vi "seq analyse.vi"(0 "config":T1={"initialize"=enum."SR830", "6221"={"6221 Resource"="GPIB0::24::INSTR", "Delta status"=FALSE, "电流|RMS(A)"=0.0}, "SR830+6221"={"source"=0, "Current(A)"=0.0, "阻抗(Ohm)"=0.0, "SR830 1"=FALSE, "SR830 2"=FALSE, "SR830 3"=FALSE, "SR830 4"=FALSE, "VISA 1"="", "VISA 2"="", "VISA 3"="", "VISA 4"="", "Reserve 1"=-1, "Reserve 2"=-1, "Reserve 3"=-1, "Reserve 4"=-1, "Sensitivity 1"=-1, "Sensitivity 2"=-1, "Sensitivity 3"=-1, "Sensitivity 4"=-1, "量程入 1"=0, "量程入 2"=0, "量程入 3"=0, "量程入 4"=0}, "2400"={"2400"=FALSE, "VISA"="GPIB0::9::INSTR", "Output Level (0)"=1e-05, "Compliance  Level (0.1)"=10.0, "ch"=[]}, "ch"={"ch"=[], "current"=[], "change?"=[], "holding current\nwhen change ch?"=FALSE, "current offset"=[]}, "Instrument"={"limit"={"Field limit"=0.0, "Field rate limit"=0.0, "Temp limit"=0.0, "Temp low limit"=0.0, "Temp rate limit "=0.0}, "genarl"={"行数"=refnum, "编辑列表框？"=refnum, "列表框"=refnum, "camg 振荡状态"=refnum, "Aborting"=refnum, "数据文件"=refnum, "warning"=refnum, "vi路径"="", "Instrument Type"=enum."PPMS-Rotate"}, "cmag"={"TM620"="TCPIP0::192.168.1.5::4266::SOCKET", "M24C Resource"="GPIB0::24::INSTR", "4G supply"="", "Temp Status 24C"=refnum, "Temp"=refnum, "9T信号"=refnum, "4g supply status"=refnum, "in-plane"="", "out-plane"="", "in-plane signal"=FALSE, "out-plane signal"=FALSE, "in plane 信号"=refnum, "pzt volt"=refnum, "camg Rate"=refnum}, "lengtou2"={"750 visa"="", "750 rotate"="", "semaphore 340"=refnum, "semaphore 750"=refnum, "750 field status"=refnum, "Input (0:A) 340"=0, "340 Resource"="GPIB0::14::INSTR", "340 Status"=refnum, "Input (0:B) 340"=1, "Loop (0: 1)"=0, "Loop (1: 1)"=0, "TCP master instance"=refnum}, "lengtou"={"TCP master instance"=refnum, "335 Status"=refnum, "335 Resource "="GPIB0::24::INSTR", "Input (0:A) 335"=0, "Input (0:B) 335"=1, "Heater Output (1:1) 335"=1, "semaphore 335"=refnum}, "325 for test"={"quantum design"=refnum, "semaphore 325"=refnum, "325 Resource "="GPIB0::13::INSTR", "Input (0:A) 325"=0, "Heater Output (1:1) 325"=1, "325 Status"=refnum}}, "2614B"={"2614B chA"=FALSE, "2614B chB"=FALSE, "VISA"=""}, "33522b"={"33522b resource name"="GPIB0::16::INSTR", "零电压"=0.0, "最大电压"=148.0, "间隔"=4.0, "最小电压"=-48.0, "loop"=0.0, "压电陶瓷电压(Vpp)"=0.0}, "gating type"=enum."2614(daul)", "层数"=0, "行数"=0, "是否处理"=[], "current 2"=[], "StrainCell"={"RP100 resource name"="GPIB0::16::INSTR", "E4980 resource name"="GPIB0::16::INSTR", "RP100 Reset ?(True)"=TRUE, "Voltage1(V)"=0.0, "Voltage2(V)"=148.0, "interval"=4.0, "slew(V/s)"=-48.0}} {"Instrument"."325 for test"."Heater Output (1:1) 325" items=["1"=1, "2"=2]; "Instrument"."325 for test"."Input (0:A) 325" items=["A", "B"]; "Instrument"."lengtou"."Heater Output (1:1) 335" items=["1"=1, "2"=2]; "Instrument"."lengtou"."Input (0:B) 335" items=["A", "B"]; "Instrument"."lengtou"."Input (0:A) 335" items=["A", "B"]; "Instrument"."lengtou2"."Loop (1: 1)" items=["1", "2"]; "Instrument"."lengtou2"."Loop (0: 1)" items=["1", "2"]; "Instrument"."lengtou2"."Input (0:B) 340" items=["A", "B", "C", "D"]; "Instrument"."lengtou2"."Input (0:A) 340" items=["A", "B", "C", "D"]; "SR830+6221"."Sensitivity 4" items=["Auto Gain"=-1, "2 nV/fA"=0, "5 nV/fA"=1, "10 nV/fA"=2, "20 nV/fA"=3, "50 nV/fA"=4, "100 nV/fA"=5, "200 nV/fA"=6, "500 nV/fA"=7, "1 uV/pA"=8, "2 uV/pA"=9, "5 uV/pA"=10, "10 uV/pA"=11, "20 uV/pA"=12, "50 uV/pA"=13, "100 uV/pA"=14, "200 uV/pA"=15, "500 uV/pA"=16, "1 mV/nA"=17, "2 mV/nA"=18, "5 mV/nA"=19, "10 mV/nA"=20, "20 mV/nA"=21, "50 mV/nA"=22, "100 mV/nA"=23, "200 mV/nA"=24, "500 mV/mA"=25, "1 V/uA"=26]; "SR830+6221"."Sensitivity 3" items=["Auto Gain"=-1, "2 nV/fA"=0, "5 nV/fA"=1, "10 nV/fA"=2, "20 nV/fA"=3, "50 nV/fA"=4, "100 nV/fA"=5, "200 nV/fA"=6, "500 nV/fA"=7, "1 uV/pA"=8, "2 uV/pA"=9, "5 uV/pA"=10, "10 uV/pA"=11, "20 uV/pA"=12, "50 uV/pA"=13, "100 uV/pA"=14, "200 uV/pA"=15, "500 uV/pA"=16, "1 mV/nA"=17, "2 mV/nA"=18, "5 mV/nA"=19, "10 mV/nA"=20, "20 mV/nA"=21, "50 mV/nA"=22, "100 mV/nA"=23, "200 mV/nA"=24, "500 mV/mA"=25, "1 V/uA"=26]; "SR830+6221"."Sensitivity 1" items=["Auto Gain"=-1, "2 nV/fA"=0, "5 nV/fA"=1, "10 nV/fA"=2, "20 nV/fA"=3, "50 nV/fA"=4, "100 nV/fA"=5, "200 nV/fA"=6, "500 nV/fA"=7, "1 uV/pA"=8, "2 uV/pA"=9, "5 uV/pA"=10, "10 uV/pA"=11, "20 uV/pA"=12, "50 uV/pA"=13, "100 uV/pA"=14, "200 uV/pA"=15, "500 uV/pA"=16, "1 mV/nA"=17, "2 mV/nA"=18, "5 mV/nA"=19, "10 mV/nA"=20, "20 mV/nA"=21, "50 mV/nA"=22, "100 mV/nA"=23, "200 mV/nA"=24, "500 mV/mA"=25, "1 V/uA"=26]; "SR830+6221"."Sensitivity 2" items=["Auto Gain"=-1, "2 nV/fA"=0, "5 nV/fA"=1, "10 nV/fA"=2, "20 nV/fA"=3, "50 nV/fA"=4, "100 nV/fA"=5, "200 nV/fA"=6, "500 nV/fA"=7, "1 uV/pA"=8, "2 uV/pA"=9, "5 uV/pA"=10, "10 uV/pA"=11, "20 uV/pA"=12, "50 uV/pA"=13, "100 uV/pA"=14, "200 uV/pA"=15, "500 uV/pA"=16, "1 mV/nA"=17, "2 mV/nA"=18, "5 mV/nA"=19, "10 mV/nA"=20, "20 mV/nA"=21, "50 mV/nA"=22, "100 mV/nA"=23, "200 mV/nA"=24, "500 mV/mA"=25, "1 V/uA"=26]; "SR830+6221"."Reserve 4" items=["Auto Reserve"=-1, "High Reserve"=0, "Normal"=1, "Low Noise"=2]; "SR830+6221"."Reserve 3" items=["Auto Reserve"=-1, "High Reserve"=0, "Normal"=1, "Low Noise"=2]; "SR830+6221"."Reserve 2" items=["Auto Reserve"=-1, "High Reserve"=0, "Normal"=1, "Low Noise"=2]; "SR830+6221"."Reserve 1" items=["Auto Reserve"=-1, "High Reserve"=0, "Normal"=1, "Low Noise"=2]; "SR830+6221"."source" items=["SR830 1", "SR830 2", "SR830 3", "SR830 4"]}, 2 "数据队列":refnum<queue>, 3 "错误输入":errorcluster) -> (7 "config out":T1={"initialize"=enum."SR830", "6221"={"6221 Resource"="GPIB0::24::INSTR", "Delta status"=FALSE, "电流|RMS(A)"=0.0}, "SR830+6221"={"source"=0, "Current(A)"=0.0, "阻抗(Ohm)"=0.0, "SR830 1"=FALSE, "SR830 2"=FALSE, "SR830 3"=FALSE, "SR830 4"=FALSE, "VISA 1"="", "VISA 2"="", "VISA 3"="", "VISA 4"="", "Reserve 1"=-1, "Reserve 2"=-1, "Reserve 3"=-1, "Reserve 4"=-1, "Sensitivity 1"=-1, "Sensitivity 2"=-1, "Sensitivity 3"=-1, "Sensitivity 4"=-1, "量程入 1"=0, "量程入 2"=0, "量程入 3"=0, "量程入 4"=0}, "2400"={"2400"=FALSE, "VISA"="GPIB0::9::INSTR", "Output Level (0)"=1e-05, "Compliance  Level (0.1)"=10.0, "ch"=[]}, "ch"={"ch"=[], "current"=[], "change?"=[], "holding current\nwhen change ch?"=FALSE, "current offset"=[]}, "Instrument"={"limit"={"Field limit"=0.0, "Field rate limit"=0.0, "Temp limit"=0.0, "Temp low limit"=0.0, "Temp rate limit "=0.0}, "genarl"={"行数"=refnum, "编辑列表框？"=refnum, "列表框"=refnum, "camg 振荡状态"=refnum, "Aborting"=refnum, "数据文件"=refnum, "warning"=refnum, "vi路径"="", "Instrument Type"=enum."PPMS-Rotate"}, "cmag"={"TM620"="TCPIP0::192.168.1.5::4266::SOCKET", "M24C Resource"="GPIB0::24::INSTR", "4G supply"="", "Temp Status 24C"=refnum, "Temp"=refnum, "9T信号"=refnum, "4g supply status"=refnum, "in-plane"="", "out-plane"="", "in-plane signal"=FALSE, "out-plane signal"=FALSE, "in plane 信号"=refnum, "pzt volt"=refnum, "camg Rate"=refnum}, "lengtou2"={"750 visa"="", "750 rotate"="", "semaphore 340"=refnum, "semaphore 750"=refnum, "750 field status"=refnum, "Input (0:A) 340"=0, "340 Resource"="GPIB0::14::INSTR", "340 Status"=refnum, "Input (0:B) 340"=1, "Loop (0: 1)"=0, "Loop (1: 1)"=0, "TCP master instance"=refnum}, "lengtou"={"TCP master instance"=refnum, "335 Status"=refnum, "335 Resource "="GPIB0::24::INSTR", "Input (0:A) 335"=0, "Input (0:B) 335"=1, "Heater Output (1:1) 335"=1, "semaphore 335"=refnum}, "325 for test"={"quantum design"=refnum, "semaphore 325"=refnum, "325 Resource "="GPIB0::13::INSTR", "Input (0:A) 325"=0, "Heater Output (1:1) 325"=1, "325 Status"=refnum}}, "2614B"={"2614B chA"=FALSE, "2614B chB"=FALSE, "VISA"=""}, "33522b"={"33522b resource name"="GPIB0::16::INSTR", "零电压"=0.0, "最大电压"=148.0, "间隔"=4.0, "最小电压"=-48.0, "loop"=0.0, "压电陶瓷电压(Vpp)"=0.0}, "gating type"=enum."2614(daul)", "层数"=0, "行数"=0, "是否处理"=[], "current 2"=[], "StrainCell"={"RP100 resource name"="GPIB0::16::INSTR", "E4980 resource name"="GPIB0::16::INSTR", "RP100 Reset ?(True)"=TRUE, "Voltage1(V)"=0.0, "Voltage2(V)"=148.0, "interval"=4.0, "slew(V/s)"=-48.0}} {"Instrument"."325 for test"."Heater Output (1:1) 325" items=["1"=1, "2"=2]; "Instrument"."325 for test"."Input (0:A) 325" items=["A", "B"]; "Instrument"."lengtou"."Heater Output (1:1) 335" items=["1"=1, "2"=2]; "Instrument"."lengtou"."Input (0:B) 335" items=["A", "B"]; "Instrument"."lengtou"."Input (0:A) 335" items=["A", "B"]; "Instrument"."lengtou2"."Loop (1: 1)" items=["1", "2"]; "Instrument"."lengtou2"."Loop (0: 1)" items=["1", "2"]; "Instrument"."lengtou2"."Input (0:B) 340" items=["A", "B", "C", "D"]; "Instrument"."lengtou2"."Input (0:A) 340" items=["A", "B", "C", "D"]; "SR830+6221"."Sensitivity 4" items=["Auto Gain"=-1, "2 nV/fA"=0, "5 nV/fA"=1, "10 nV/fA"=2, "20 nV/fA"=3, "50 nV/fA"=4, "100 nV/fA"=5, "200 nV/fA"=6, "500 nV/fA"=7, "1 uV/pA"=8, "2 uV/pA"=9, "5 uV/pA"=10, "10 uV/pA"=11, "20 uV/pA"=12, "50 uV/pA"=13, "100 uV/pA"=14, "200 uV/pA"=15, "500 uV/pA"=16, "1 mV/nA"=17, "2 mV/nA"=18, "5 mV/nA"=19, "10 mV/nA"=20, "20 mV/nA"=21, "50 mV/nA"=22, "100 mV/nA"=23, "200 mV/nA"=24, "500 mV/mA"=25, "1 V/uA"=26]; "SR830+6221"."Sensitivity 3" items=["Auto Gain"=-1, "2 nV/fA"=0, "5 nV/fA"=1, "10 nV/fA"=2, "20 nV/fA"=3, "50 nV/fA"=4, "100 nV/fA"=5, "200 nV/fA"=6, "500 nV/fA"=7, "1 uV/pA"=8, "2 uV/pA"=9, "5 uV/pA"=10, "10 uV/pA"=11, "20 uV/pA"=12, "50 uV/pA"=13, "100 uV/pA"=14, "200 uV/pA"=15, "500 uV/pA"=16, "1 mV/nA"=17, "2 mV/nA"=18, "5 mV/nA"=19, "10 mV/nA"=20, "20 mV/nA"=21, "50 mV/nA"=22, "100 mV/nA"=23, "200 mV/nA"=24, "500 mV/mA"=25, "1 V/uA"=26]; "SR830+6221"."Sensitivity 1" items=["Auto Gain"=-1, "2 nV/fA"=0, "5 nV/fA"=1, "10 nV/fA"=2, "20 nV/fA"=3, "50 nV/fA"=4, "100 nV/fA"=5, "200 nV/fA"=6, "500 nV/fA"=7, "1 uV/pA"=8, "2 uV/pA"=9, "5 uV/pA"=10, "10 uV/pA"=11, "20 uV/pA"=12, "50 uV/pA"=13, "100 uV/pA"=14, "200 uV/pA"=15, "500 uV/pA"=16, "1 mV/nA"=17, "2 mV/nA"=18, "5 mV/nA"=19, "10 mV/nA"=20, "20 mV/nA"=21, "50 mV/nA"=22, "100 mV/nA"=23, "200 mV/nA"=24, "500 mV/mA"=25, "1 V/uA"=26]; "SR830+6221"."Sensitivity 2" items=["Auto Gain"=-1, "2 nV/fA"=0, "5 nV/fA"=1, "10 nV/fA"=2, "20 nV/fA"=3, "50 nV/fA"=4, "100 nV/fA"=5, "200 nV/fA"=6, "500 nV/fA"=7, "1 uV/pA"=8, "2 uV/pA"=9, "5 uV/pA"=10, "10 uV/pA"=11, "20 uV/pA"=12, "50 uV/pA"=13, "100 uV/pA"=14, "200 uV/pA"=15, "500 uV/pA"=16, "1 mV/nA"=17, "2 mV/nA"=18, "5 mV/nA"=19, "10 mV/nA"=20, "20 mV/nA"=21, "50 mV/nA"=22, "100 mV/nA"=23, "200 mV/nA"=24, "500 mV/mA"=25, "1 V/uA"=26]; "SR830+6221"."Reserve 4" items=["Auto Reserve"=-1, "High Reserve"=0, "Normal"=1, "Low Noise"=2]; "SR830+6221"."Reserve 3" items=["Auto Reserve"=-1, "High Reserve"=0, "Normal"=1, "Low Noise"=2]; "SR830+6221"."Reserve 2" items=["Auto Reserve"=-1, "High Reserve"=0, "Normal"=1, "Low Noise"=2]; "SR830+6221"."Reserve 1" items=["Auto Reserve"=-1, "High Reserve"=0, "Normal"=1, "Low Noise"=2]; "SR830+6221"."source" items=["SR830 1", "SR830 2", "SR830 3", "SR830 4"]}, 10 "错误输出":errorcluster)   [LabVIEW 2019, in "User lib.lvlib"]
uses:
  User lib.lvlib
  ctl/config.ctl
  <vilib>/NI/Modbus Library/API/Master/Modbus Master.lvclass
  ctl/initialize.ctl
  ctl/Instrument.ctl
  ctl/limit.ctl
  ctl/warning.ctl
  ctl/Instrument Type.ctl
  ctl/335 state.ctl
  ctl/9T mag field stauts.ctl
  C:/Users/fuyang/Desktop/postdoctor/labview/labview-measure/lib/QDInstrument.dll
  lib/QDInstrument.dll
  ctl/Gating type.ctl
  ctl/set type.ctl
  SubVI.lvlib
  Take Seq.lvlib
  9T cmag.lvlib
  Scan.lvlib
  nematic/Copy of StrainCell.lvlib
panel:
  out "step":string
  out "数值":i32
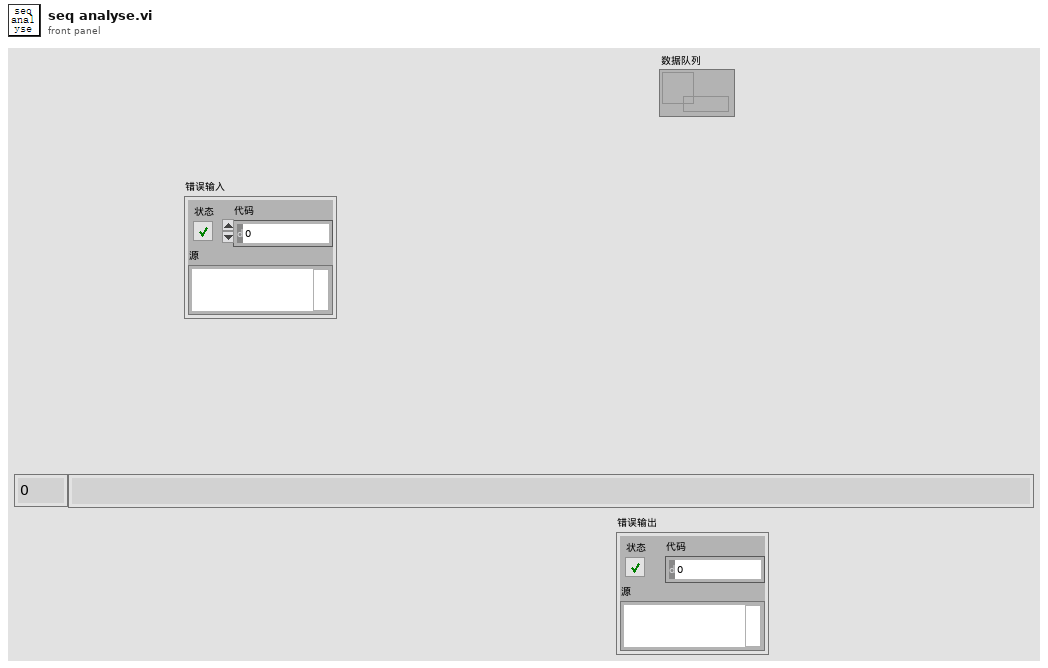
[diagram p1: front panel]
types:
  T1 = typedef "config.ctl" = cluster{"initialize":T2, "6221":cluster{"6221 Resource":refnum<visa-resource-name>, "Delta status":bool, "电流|RMS(A)":dbl}, "SR830+6221":cluster{"source":u16, "Current(A)":dbl, "阻抗(Ohm)":dbl, "SR830 1":bool, "SR830 2":bool, "SR830 3":bool, "SR830 4":bool, "VISA 1":refnum<visa-resource-name>, "VISA 2":refnum<visa-resource-name>, "VISA 3":refnum<visa-resource-name>, "VISA 4":refnum<visa-resource-name>, "Reserve 1":i16, "Reserve 2":i16, "Reserve 3":i16, "Reserve 4":i16, "Sensitivity 1":i16, "Sensitivity 2":i16, "Sensitivity 3":i16, "Sensitivity 4":i16, "量程入 1":i32, "量程入 2":i32, "量程入 3":i32, "量程入 4":i32}, "2400":cluster{"2400":bool, "VISA":refnum<visa-resource-name>, "Output Level (0)":dbl, "Compliance  Level (0.1)":dbl, "ch":i32[]}, "ch":cluster{"ch":i32[], "current":dbl[], "change?":bool[], "holding current\nwhen change ch?":bool, "current offset":dbl[]}, "Instrument":T3, "2614B":cluster{"2614B chA":bool, "2614B chB":bool, "VISA":refnum<visa-resource-name>}, "33522b":cluster{"33522b resource name":refnum<visa-resource-name>, "零电压":dbl, "最大电压":dbl, "间隔":dbl, "最小电压":dbl, "loop":dbl, "压电陶瓷电压(Vpp)":dbl}, "gating type":T7, "层数":i32, "行数":i32, "是否处理":bool[], "current 2":dbl[], "StrainCell":cluster{"RP100 resource name":refnum<visa-resource-name>, "E4980 resource name":refnum<visa-resource-name>, "RP100 Reset ?(True)":bool, "Voltage1(V)":dbl, "Voltage2(V)":dbl, "interval":dbl, "slew(V/s)":dbl}}
  T2 = typedef "initialize.ctl" = enum16{"SR830", "keithley6221-SR830", "Delta", "Delta-tunnelling", "keithley6221-2182-DC", "PZT", "StrainCell", "4200"}
  T3 = typedef "Instrument.ctl" = cluster{"limit":T4, "genarl":cluster{"行数":refnum<vi>, "编辑列表框？":refnum<vi>, "列表框":refnum<vi>, "camg 振荡状态":refnum<vi>, "Aborting":refnum<vi>, "数据文件":refnum<vi>, "warning":refnum<vi>, "vi路径":string, "Instrument Type":T5}, "cmag":cluster{"TM620":refnum<visa-resource-name>, "M24C Resource":refnum<visa-resource-name>, "4G supply":refnum<visa-resource-name>, "Temp Status 24C":refnum<vi>, "Temp":refnum<vi>, "9T信号":T6, "4g supply status":refnum<vi>, "in-plane":refnum<visa-resource-name>, "out-plane":refnum<visa-resource-name>, "in-plane signal":bool, "out-plane signal":bool, "in plane 信号":T6, "pzt volt":refnum<vi>, "camg Rate":refnum<vi>}, "lengtou2":cluster{"750 visa":refnum<visa-resource-name>, "750 rotate":refnum<visa-resource-name>, "semaphore 340":T6, "semaphore 750":T6, "750 field status":refnum<vi>, "Input (0:A) 340":u16, "340 Resource":refnum<visa-resource-name>, "340 Status":refnum<vi>, "Input (0:B) 340":u16, "Loop (0: 1)":u16, "Loop (1: 1)":u16, "TCP master instance":refnum<class "Modbus Master.lvclass">}, "lengtou":cluster{"TCP master instance":refnum<class "Modbus Master.lvclass">, "335 Status":refnum<vi>, "335 Resource ":refnum<visa-resource-name>, "Input (0:A) 335":u16, "Input (0:B) 335":u16, "Heater Output (1:1) 335":u16, "semaphore 335":T6}, "325 for test":cluster{"quantum design":refnum<k24>, "semaphore 325":T6, "325 Resource ":refnum<visa-resource-name>, "Input (0:A) 325":u16, "Heater Output (1:1) 325":u16, "325 Status":refnum<vi>}}
  T4 = typedef "limit.ctl" = cluster{"Field limit":dbl, "Field rate limit":dbl, "Temp limit":dbl, "Temp low limit":dbl, "Temp rate limit ":dbl}
  T5 = typedef "Instrument Type.ctl" = enum16{"PPMS", "VersaLab", "DynaCool", "SVSM", "PPMS-Rotate", "Lakeshore335", "lengtou2", "9T mag old", "9T cmag", "9T cmag DAC", "9T cmag rotate", "test"}
  T6 = typedef "Semaphore RefNum" = refnum<k1>
  T7 = typedef "Gating type.ctl" = enum32{"null", "2614(daul)", "2400", "6517B"}
  T8 = typedef "set type.ctl" = enum16{"temp", "field", "position", "gating", "current", "PZT", "StrainCell", "time"}
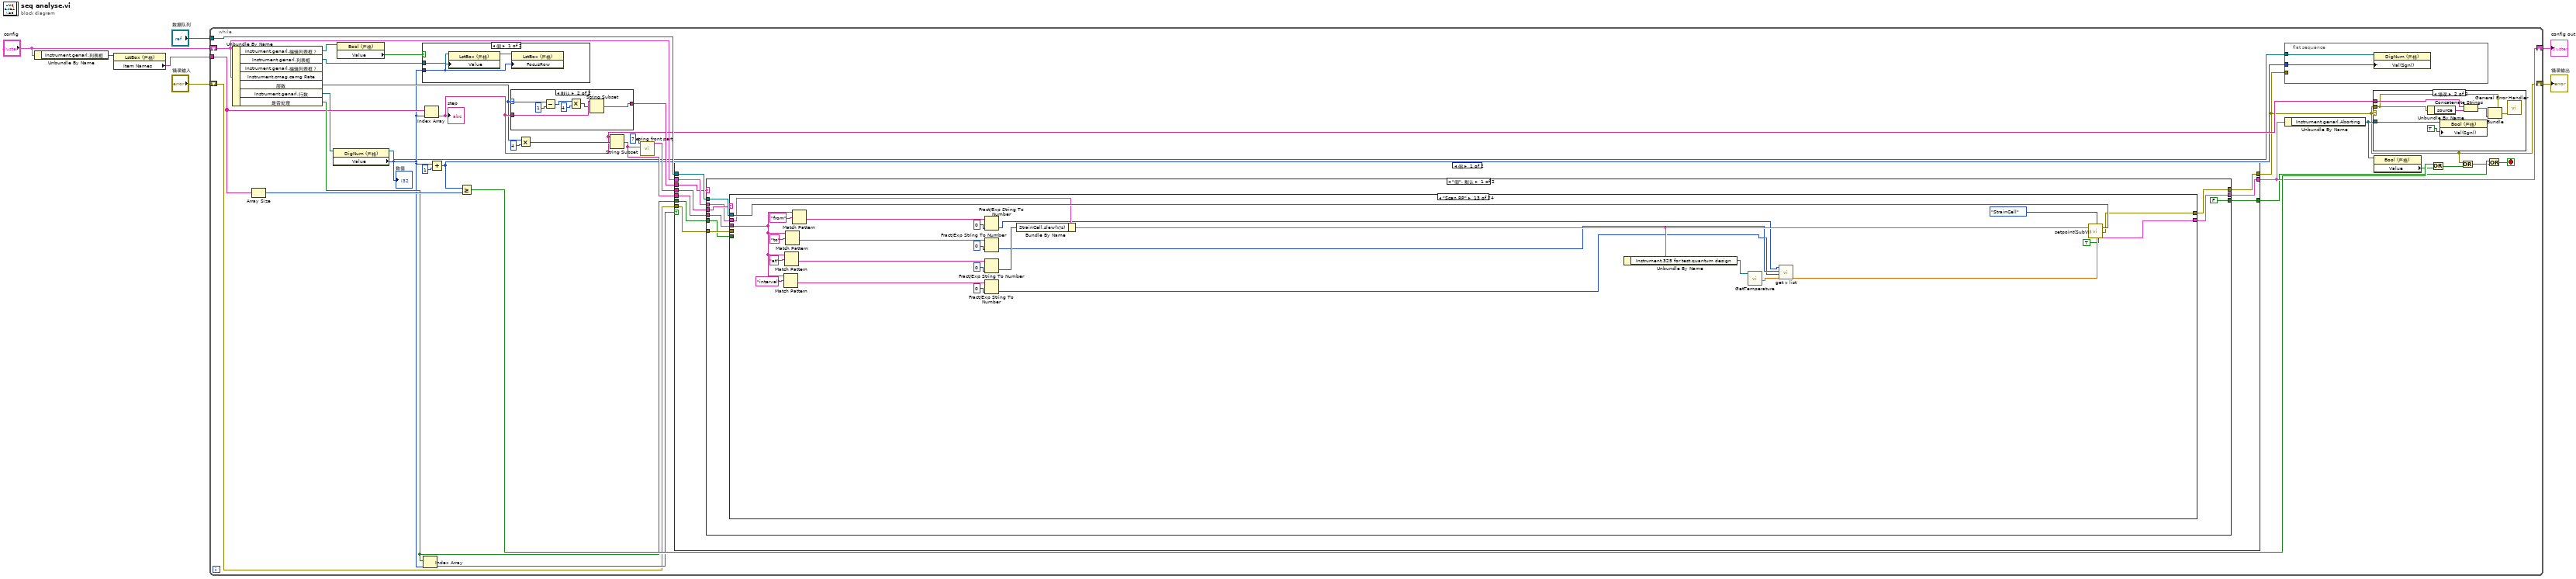
[diagram p0: block diagram]
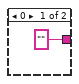
[diagram p2: hidden frame]
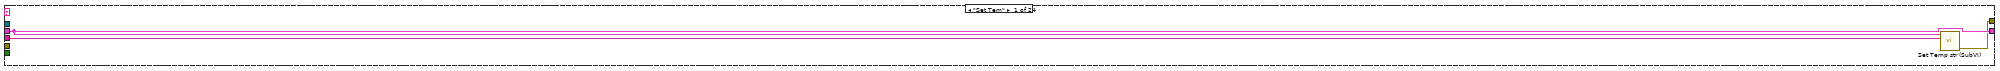
[diagram p5: hidden frame]
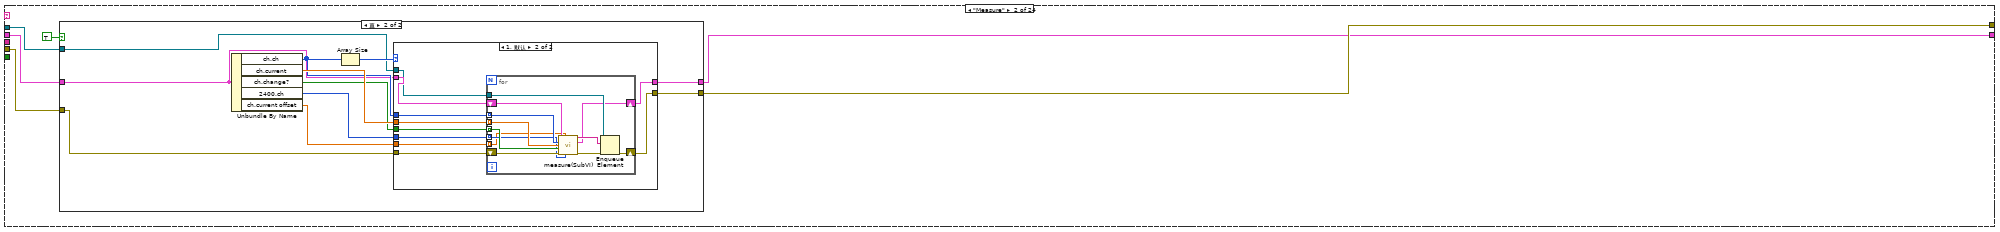
[diagram p6: hidden frame]
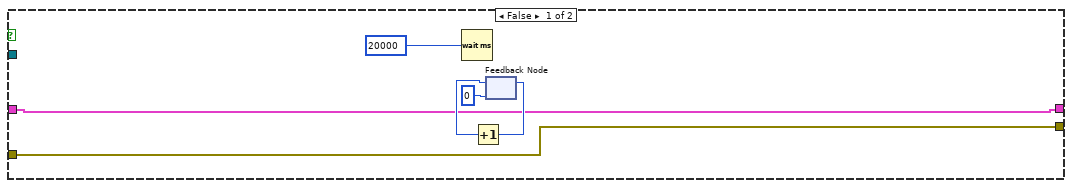
[diagram p7: hidden frame]
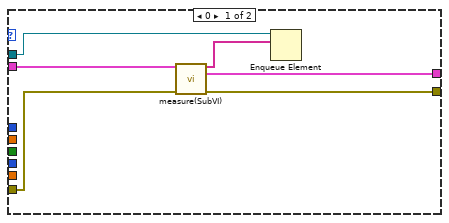
[diagram p8: hidden frame]
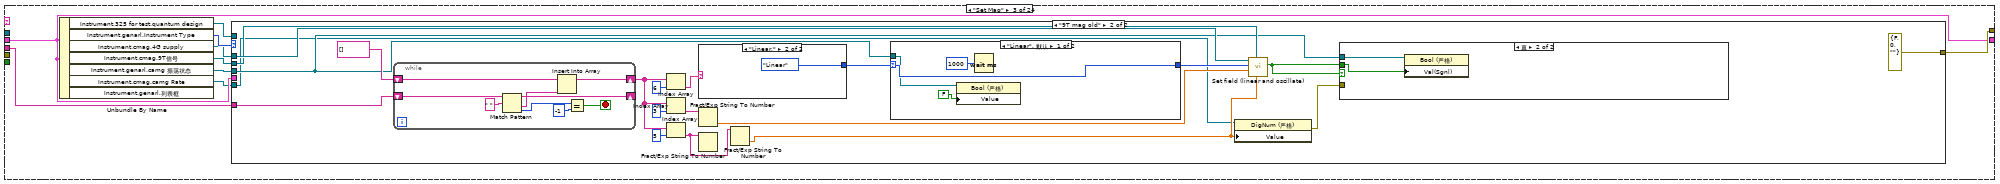
[diagram p9: hidden frame]
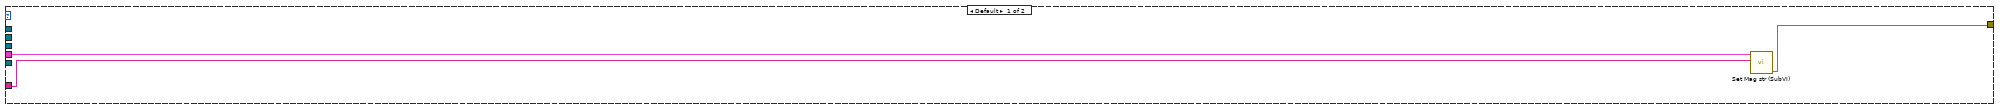
[diagram p10: hidden frame]
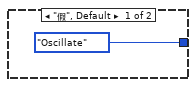
[diagram p13: hidden frame]
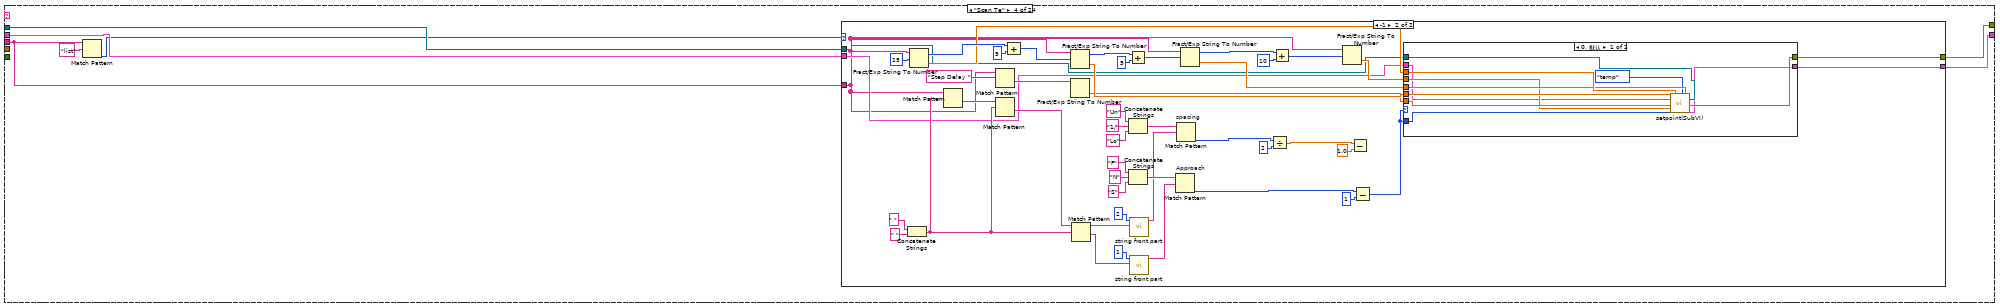
[diagram p14: hidden frame]
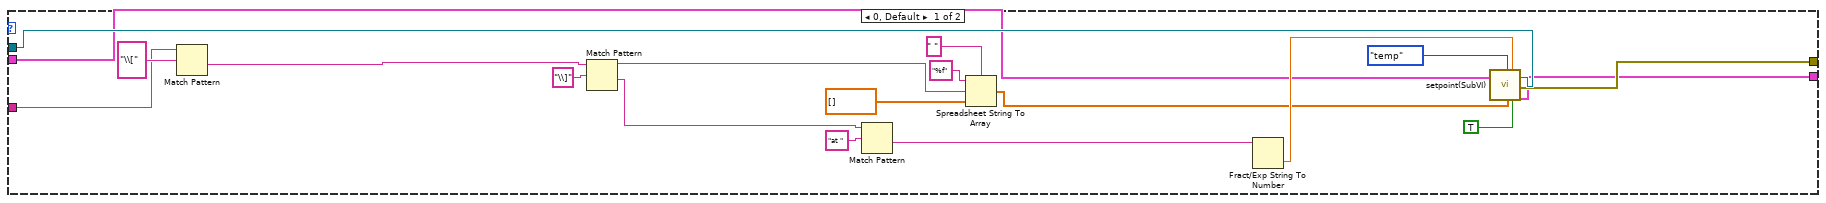
[diagram p15: hidden frame]
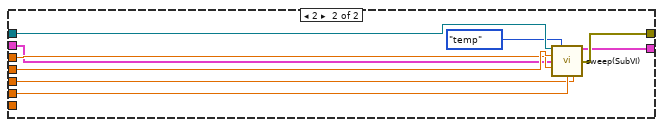
[diagram p16: hidden frame]
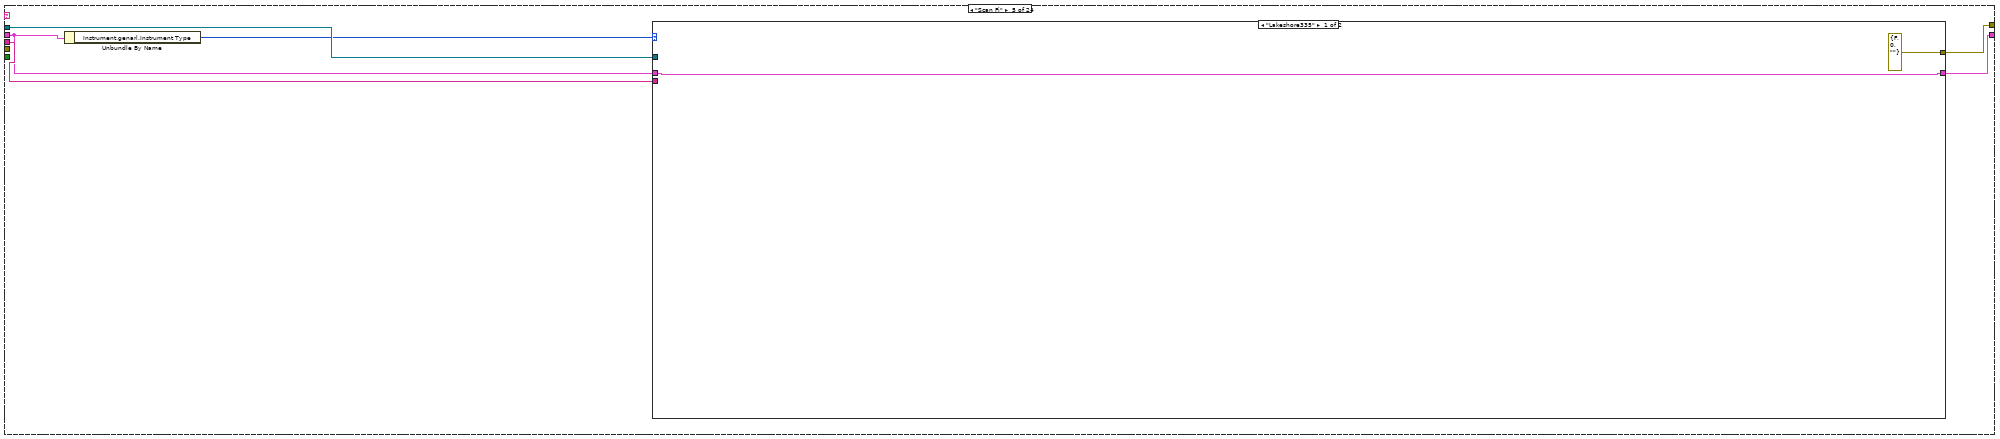
[diagram p17: hidden frame]
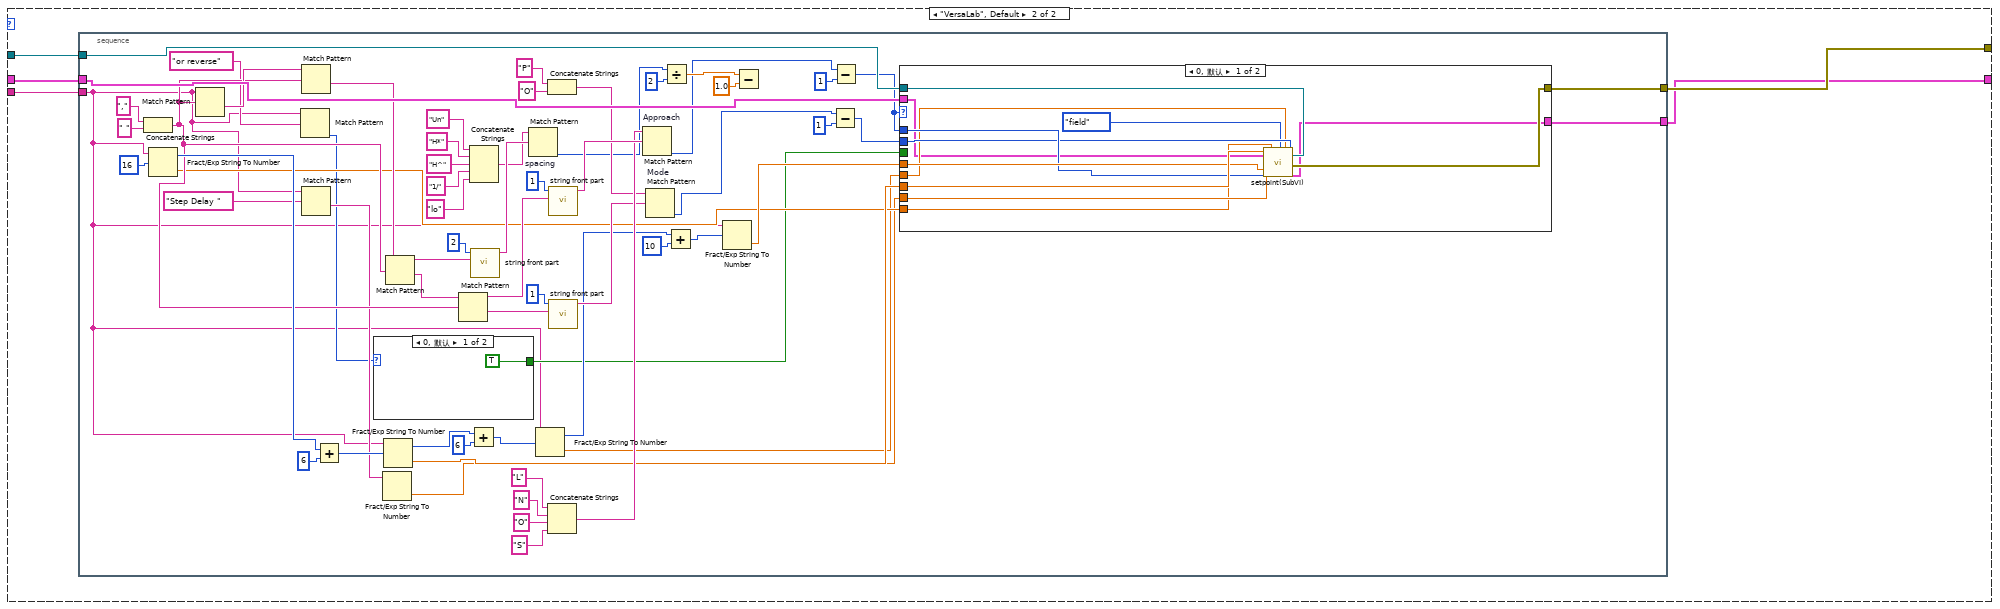
[diagram p18: hidden frame]
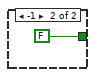
[diagram p19: hidden frame]
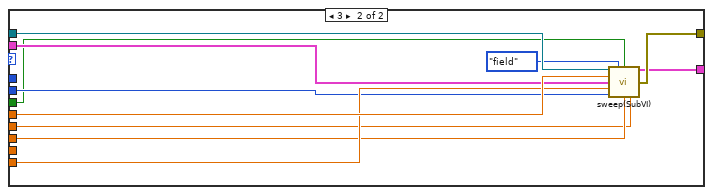
[diagram p20: hidden frame]
diagram:
  n1 = Unbundle By Name("config") -> ("Instrument.genarl.列表框"=w2:refnum<vi>)
  n2 = property class="LstBox (严格)"(reference=w2) -> ("Item Names"=w4:string[])  [unwired: 1 in, 2 out]
  n3 = while {
    tunnel: "数据队列" -> [w38]
    shift-right: [w33] -> w5
    shift-left: "config" -> [w11]
    tunnel: w4 -> [w14]
    shift-right: [w8] -> w1
    shift-left: "错误输入" -> [w22]
    stop <- w25 stop-if-true
    n4 = Unbundle By Name(w11) -> ("Instrument.genarl.编辑列表框？"=w21:refnum<vi>, "Instrument.genarl.列表框"=w18:refnum<vi>, "层数"=w16:i32, "Instrument.genarl.行数"=w13:refnum<vi>, "是否处理"=w15:bool[])  [unwired: 2 out]
    n5 = Array Size(array=w14) -> (size(s)=w24:i32)
    n6 = property class="DigNum (严格)"(reference=w13) -> (reference out=w10:refnum<vi>, "Value"=w12:i32)  [unwired: 1 in, 1 out]
    "数值" <- w12
    n7 = property class="Bool (严格)"(reference=w21) -> ("Value"=w20:bool)  [unwired: 1 in, 2 out]
    n8 = case shown="假" w20 {
      tunnel: w12 -> [w59 _]
      tunnel: w18 -> [w57 _]
      frame False {
        n9 = property on="属性节点" class="LstBox (严格)"(reference=w57, "Value"=w59) -> (reference out=w58:refnum<vi>)  [unwired: 1 in, 1 out]
        n10 = property on="属性节点" class="LstBox (严格)"(reference=w58, "FocusRow"=w59) -> ()  [unwired: 1 in, 2 out]
      }
      frame True {
      }
    }
    n11 = Index Array(array=w15, index=w12) -> (element=w36:bool)
    n12 = Index Array(array=w14, index=w12) -> (element=w17:string)
    "step" <- w17
    n13 = Add(x=w12, y=1) -> (x+y=w9:i32)
    n14 = Greater Or Equal?(x=w9, y=w24) -> (x >= y?=w37:bool)
    n15 = case shown="默认" w16 {
      selector: w16 -> [_ w49]
      tunnel: w17 -> [_ w46]
      tunnel: ["" w43] -> w30
      frame 0 {
      }
      frame Default {
        n16 = Subtract(x=w49, y=1) -> (x-y=w47:i32)
        n17 = Multiply(x=w47, y=4) -> (x*y=w44:i32)
        n18 = String Subset(string=w46, offset (0)=w44) -> (substring=w43:string)  [unwired: 1 in]
      }
    }
    n19 = Multiply(x=w16, y=4) -> (x*y=w28:i32)
    n20 = String Subset(string=w17, offset (0)=w28) -> (substring=w19:string)  [unwired: 1 in]
    n21 = call "string front part.vi"("字符串"=w19, "偏移量(0)"=7 ("y")) -> ("result string"=w34:string)  [unwired: 9 in]
    n22 = case shown="假" w36 {
      tunnel: w19 -> [w69 _]
      tunnel: w38 -> [w68 _]
      tunnel: w34 -> [w67 _]
      tunnel: [w64 errorcluster {"status"=FALSE, "code"=0, "source"=""} ("错误输出")] -> w8
      tunnel: w11 -> [w66 w661]
      tunnel: [w65 w661] -> w33
      tunnel: w30 -> [w63 _]
      tunnel: [w62 FALSE] -> w27
      tunnel: w22 -> [w61 _]
      tunnel: w15 -> [w60 _]
      frame False {
        n23 = case shown="\"假\", 默认" w63 {
          tunnel: w69 -> [w78 _]
          tunnel: w68 -> [w77 _]
          tunnel: w67 -> [w76 _]
          tunnel: w66 -> [w75 w657]
          tunnel: [w74 w657] -> w65
          tunnel: [w73 errorcluster {"status"=FALSE, "code"=0, "source"=""} ("错误输出")] -> w64
          tunnel: [FALSE TRUE] -> w62
          tunnel: w61 -> [w71 _]
          tunnel: w60 -> [w70 _]
          frame "假", Default {
            n24 = case shown="\"Scan RP\"" w76 {
              tunnel: w78 -> [w81 _ w141 w184 w281 w382 _ w389 w394 _ w402 w404 w434 w453 w464 w468 w471 w477 w564 w577 w581 w613 w632 _]
              tunnel: w77 -> [_ w87 _ w186 w282 _ _ _ _ _ _ w403 w441 _ w465 _ _ w476 _ _ w582 _ w623 _]
              tunnel: w75 -> [w80 w86 w135 w189 w278 w381 w384 w387 w392 w396 w399 w419 w433 w452 w463 w467 w470 w473 w560 w576 w579 w611 w624 w656]
              tunnel: [w80 w82 w135 w187 w279 w380 w384 w387 w392 w396 w401 w418 w440 w451 w462 w467 w470 w474 w560 w575 w580 w611 w622 w656] -> w74
              tunnel: [w79 w84 w136 w188 w277 errorcluster {"status"=FALSE, "code"=0, "source"=""} ("错误输出") errorcluster {"status"=FALSE, "code"=0, "source"=""} ("错误输出") w386 w393 errorcluster {"status"=FALSE, "code"=0, "source"=""} ("错误输出") errorcluster {"status"=FALSE, "code"=0, "source"=""} ("错误输出") w417 w439 w450 w461 w466 w469 w472 w561 errorcluster {"status"=FALSE, "code"=0, "source"=""} ("错误输出") w578 w608 w621 errorcluster {"status"=FALSE, "code"=0, "source"=""} ("错误输出")] -> w73
              tunnel: w71 -> [_ w85 _ _ _ _ w383 _ _ _ _ _ _ w449 _ _ _ _ _ _ _ _ _ _]
              tunnel: w70 -> [_ _ _ _ _ _ _ _ _ _ _ _ _ _ _ _ _ _ _ _ _ _ _ _]
              frame "Set Tem" {
                n25 = call "Set Temp str (SubVI).vi"("字符串"=w81, "簇"=w80) -> ("错误输出"=w79:errorcluster)  [unwired: 9 in]
              }
              frame "Measure" {
                n26 = case shown="真" TRUE {
                  tunnel: w87 -> [_ w100]
                  tunnel: w86 -> [w89 w99]
                  tunnel: w85 -> [w93 w98]
                  tunnel: [w93 w97] -> w84
                  tunnel: [w89 w96] -> w82
                  frame False {
                    n27 = Wait (ms)(milliseconds to wait=u32 20000 ("等待时间（毫秒）")) -> ()  [unwired: 1 out]
                    n28 = feedback #1(0) -> (w91:i32)
                    n29 = Increment(x=w91) -> (x+1=w92:i32)
                    n30 = feedback-in #1(w92) -> ()
                  }
                  frame True {
                    n31 = Unbundle By Name(w99) -> ("ch.ch"=w102:i32[], "ch.current"=w104:dbl[], "ch.change?"=w103:bool[], "2400.ch"=w95:i32[], "ch.current offset"=w94:dbl[])
                    n32 = Array Size(array=w102) -> (size(s)=w101:i32)
                    n33 = case shown="1, 默认" w101 {
                      tunnel: w99 -> [w110 w120]
                      tunnel: w102 -> [_ w119]
                      tunnel: w104 -> [_ w118]
                      tunnel: w103 -> [_ w117]
                      tunnel: w100 -> [w105 w116]
                      tunnel: w98 -> [w109 w115]
                      tunnel: [w108 w114] -> w97
                      tunnel: [w107 w113] -> w96
                      tunnel: w95 -> [_ w112]
                      tunnel: w94 -> [_ w111]
                      frame 0 {
                        n34 = call "measure(SubVI).vi"("config in"=w110, "error in (no error)"=w109) -> ("data"=w106:string[], "config out"=w107:T1, "error out"=w108:errorcluster)  [unwired: 11 in]
                        n35 = Enqueue Element(queue=w105, element=w106) -> ()  [unwired: 2 in, 3 out]
                      }
                      frame 1, Default {
                        n36 = for {
                          tunnel: w119 -> [w130] mode=indexing
                          tunnel: w117 -> [w128] mode=indexing
                          tunnel: w118 -> [w129] mode=indexing
                          tunnel: w116 -> [w132]
                          shift-right: [w126] -> w113
                          shift-left: w120 -> [w131]
                          shift-right: [w123] -> w114
                          shift-left: w115 -> [w125]
                          tunnel: w112 -> [w122] mode=indexing
                          tunnel: w111 -> [w121] mode=indexing
                          n37 = call "measure(SubVI).vi"("config in"=w131, "current offset"=w121, "ch"=w130, "current"=w129, "change?"=w128, "error in (no error)"=w125, "2400ch"=w122) -> ("data"=w127:string[], "config out"=w126:T1, "error out"=w124:errorcluster)  [unwired: 6 in]
                          n38 = Enqueue Element(queue=w132, element=w127, error in (no error)=w124) -> (error out=w123:errorcluster)  [unwired: 1 in, 2 out]
                        }
                      }
                    }
                  }
                }
              }
              frame "Set Mag" {
                n39 = Unbundle By Name(w135) -> ("Instrument.325 for test.quantum design"=w140:refnum<k24>, "Instrument.genarl.Instrument Type"=w139:T5, "Instrument.cmag.4G supply"=w138:refnum<visa-resource-name>, "Instrument.cmag.9T信号"=w137:T6, "Instrument.genarl.camg 振荡状态"=w134:refnum<vi>, "Instrument.cmag.camg Rate"=w133:refnum<vi>)  [unwired: 1 out]
                n40 = case shown="\"9T mag old\"" w139 {
                  tunnel: w141 -> [w144 w163]
                  tunnel: [w143 errorcluster {"status"=FALSE, "code"=0, "source"=""} ("错误输出")] -> w136
                  tunnel: w140 -> [_ _]
                  tunnel: w138 -> [_ w153]
                  tunnel: w137 -> [_ w147]
                  tunnel: w135 -> [w142 _]
                  tunnel: w134 -> [_ w146]
                  tunnel: w133 -> [_ w145]
                  frame Default {
                    n41 = call "Set Mag str (SubVI).vi"("字符串"=w144, "输出簇输入"=w142) -> ("错误输出"=w143:errorcluster)  [unwired: 9 in]
                  }
                  frame "9T mag old" {
                    n42 = while {
                      shift-right: [w178] -> w158
                      shift-left: string[] [] -> [w177]
                      shift-right: [w180] -> _
                      shift-left: w163 -> [w182]
                      stop <- w174 stop-if-true
                      n43 = Match Pattern(string=w182, regular expression=" " ("正则表达式")) -> (before substring=w179:string, after substring=w180:string, offset past match=w176:i32)  [unwired: 1 in, 1 out]
                      n44 = Insert Into Array(array=w177, new element=w179) -> (w178:string[])  [unwired: 1 in]
                      n45 = Equal?(x=w176, y=-1) -> (x = y?=w174:bool)
                    }
                    n46 = Index Array(array=w158, index=6 ("索引")) -> (element=w155:string)
                    n47 = Index Array(array=w158, index=3 ("索引")) -> (element=w159:string)
                    n48 = Index Array(array=w158, index=5 ("索引")) -> (element=w156:string)
                    n49 = case shown="\"Linear,\"" w155 {
                      tunnel: [enum16{"Linear", "Oscillate"}."Oscillate" ("Approach") enum16{"Linear", "Oscillate"}."Linear" ("Approach")] -> w154
                      frame "假", Default {
                      }
                      frame "Linear," {
                      }
                    }
                    n50 = Fract/Exp String To Number(string=w159) -> (number=w148:dbl)  [unwired: 3 in, 1 out]
                    n51 = Fract/Exp String To Number(string=w156) -> ()  [unwired: 3 in, 2 out]
                    n52 = Fract/Exp String To Number(string=w156) -> (number=w149:dbl)  [unwired: 3 in, 1 out]
                    n53 = case shown="\"Linear\", 默认" w154 {
                      selector: w154 -> [w166 w169]
                      tunnel: [w166 w169] -> w152
                      tunnel: w146 -> [w165 _]
                      frame "Linear", Default {
                        n54 = property on="属性节点" class="Bool (严格)"(reference=w165, "Value"=FALSE ("oscillating")) -> ()  [unwired: 1 in, 2 out]
                        n55 = Wait (ms)(milliseconds to wait=u32 1000) -> ()  [unwired: 1 out]
                      }
                      frame "Oscillate" {
                      }
                    }
                    n56 = property on="属性节点" class="DigNum (严格)"(reference=w145, "Value"=w149) -> (error out=w150:errorcluster)  [unwired: 1 in, 1 out]
                    n57 = call "Set field (linear and oscillate).vi"("Rate(Oe/s)"=w149, "semaphore"=w147, "数值"=w148, "Approach"=w152, "VISA Resource Name"=w153) -> ("Oscillate?"=w151:bool)  [unwired: 3 in, 3 out]
                    n58 = case shown="真" w151 {
                      tunnel: w151 -> [_ w171]
                      tunnel: w150 -> [_ _]
                      tunnel: w146 -> [_ w170]
                      frame False {
                      }
                      frame True {
                        n59 = property on="属性节点" class="Bool (严格)"(reference=w170, "Val(Sgnl)"=w171) -> ()  [unwired: 1 in, 2 out]
                      }
                    }
                  }
                }
              }
              frame "Scan Te" {
                n60 = Match Pattern(string=w184, regular expression="list" ("正则表达式")) -> (offset past match=w183:i32)  [unwired: 1 in, 3 out]
                n61 = case shown="-1" w183 {
                  tunnel: w186 -> [w194 w210]
                  tunnel: w189 -> [w190 w230]
                  tunnel: w184 -> [w191 w209]
                  tunnel: [w193 w212] -> w188
                  tunnel: [w192 w211] -> w187
                  frame 0, Default {
                    n62 = Match Pattern(string=w191, regular expression="\\[" ("正则表达式")) -> (after substring=w206:string)  [unwired: 1 in, 3 out]
                    n63 = Match Pattern(string=w206, regular expression="\\]" ("正则表达式")) -> (before substring=w204:string, after substring=w201:string)  [unwired: 1 in, 2 out]
                    n64 = Match Pattern(string=w201, regular expression="at " ("正则表达式")) -> (after substring=w199:string)  [unwired: 1 in, 3 out]
                    n65 = Spreadsheet String To Array(delimiter (Tab)=" " ("分隔符(Tab)"), format string="%f" ("格式字符串"), spreadsheet string=w204, array type (2D Dbl)=dbl[] []) -> (array=w196:dbl[])
                    n66 = Fract/Exp String To Number(string=w199) -> (number=w198:dbl)  [unwired: 3 in, 1 out]
                    n67 = call "setpoint(SubVI).vi"("输出簇 2"=w190, "type"=set_type."temp", "list"=w196, "Rate/speed"=w198, "list?"=TRUE, "data"=w194) -> ("错误输出"=w193:errorcluster, "输出簇"=w192:T1)  [unwired: 12 in]
                  }
                  frame -1 {
                    n68 = Concatenate Strings("," ("字符串"), " " ("字符串")) -> (w246:string)
                    n69 = Fract/Exp String To Number(string=w209, offset=15 ("偏移量")) -> (offset past number=w255:i32, number=w236:dbl)  [unwired: 2 in]
                    n70 = Match Pattern(string=w209, regular expression=w246) -> (after substring=w256:string)  [unwired: 1 in, 3 out]
                    n71 = Match Pattern(string=w209, regular expression="Step Delay ") -> (after substring=w233:string)  [unwired: 1 in, 3 out]
                    n72 = Match Pattern(string=w256, regular expression=w246) -> (after substring=w247:string)  [unwired: 1 in, 3 out]
                    n73 = Add(x=w255, y=5) -> (x+y=w254:i32)
                    n74 = Fract/Exp String To Number(string=w233) -> (number=w232:dbl)  [unwired: 3 in, 1 out]
                    n75 = Fract/Exp String To Number(string=w209, offset=w254) -> (offset past number=w250:i32, number=w235:dbl)  [unwired: 2 in]
                    n76 = Match Pattern(string=w247, regular expression=w246) -> (before substring=w245:string, after substring=w239:string)  [unwired: 1 in, 2 out]
                    n77 = Add(x=w250, y=5) -> (x+y=w249:i32)
                    n78 = Concatenate Strings("Un" ("字符串"), "1/" ("字符串"), "Lo" ("字符串")) -> (w243:string)
                    n79 = Concatenate Strings("F" ("字符串"), "N" ("字符串"), "S" ("字符串")) -> (w252:string)
                    n80 = call "string front part.vi"("字符串"=w245, "偏移量(0)"=2) -> ("result string"=w244:string)  [unwired: 9 in]
                    n81 = call "string front part.vi"("字符串"=w239, "偏移量(0)"=1) -> ("result string"=w253:string)  [unwired: 9 in]
                    n82 = Match Pattern "Approach"(string=w252, regular expression=w253) -> (offset past match=w251:i32)  [unwired: 1 in, 3 out]
                    n83 = Match Pattern "spacing"(string=w243, regular expression=w244) -> (offset past match=w242:i32)  [unwired: 1 in, 3 out]
                    n84 = Fract/Exp String To Number(string=w209, offset=w249) -> (offset past number=w240:i32, number=w234:dbl)  [unwired: 2 in]
                    n85 = Divide(x=w242, y=2) -> (x/y=w241:dbl)
                    n86 = Add(x=w240, y=10) -> (x+y=w248:i32)
                    n87 = Fract/Exp String To Number(string=w209, offset=w248) -> (number=w237:dbl)  [unwired: 2 in, 1 out]
                    n88 = Subtract(x=w241, y=1.0) -> ()  [unwired: 1 out]
                    n89 = Subtract(x=w251, y=1) -> (x-y=w238:i32)
                    n90 = case shown="0, 默认" w238 {
                      tunnel: w238 -> [w262 _]
                      tunnel: w237 -> [w263 w275]
                      tunnel: w234 -> [w265 w271]
                      tunnel: w236 -> [w266 w274]
                      tunnel: w235 -> [w267 w272]
                      tunnel: w210 -> [w260 w276]
                      tunnel: [w259 w270] -> w212
                      tunnel: w232 -> [w264 _]
                      tunnel: w230 -> [w258 w269]
                      tunnel: [w257 w268] -> w211
                      frame 0, Default {
                        n91 = call "setpoint(SubVI).vi"("Filed 2"=w267, "输出簇 2"=w258, "Delay"=w264, "steps number"=w263, "Approach"=w262, "Field"=w266, "type"=enum16{"temp", "field", "position"}."temp" ("类型"), "Rate/speed"=w265, "data"=w260) -> ("错误输出"=w259:errorcluster, "输出簇"=w257:T1)  [unwired: 9 in]
                      }
                      frame 2 {
                        n92 = call "sweep(SubVI).vi"("data"=w276, "类型"=enum16{"temp", "field", "position"}."temp", "steps number"=w275, "簇"=w269, "Field"=w274, "Field 2"=w272, "Rate、speed"=w271) -> ("输出簇"=w268:T1, "错误输出"=w270:errorcluster)  [unwired: 7 in]
                      }
                    }
                  }
                }
              }
              frame "Scan Fi" {
                n93 = Unbundle By Name(w278) -> ("Instrument.genarl.Instrument Type"=w280:T5)
                n94 = case shown="\"Lakeshore335\"" w280 {
                  tunnel: w282 -> [_ w289]
                  tunnel: [errorcluster {"status"=FALSE, "code"=0, "source"=""} ("错误输出") w288] -> w277
                  tunnel: w281 -> [_ w287]
                  tunnel: w278 -> [w283 w286]
                  tunnel: [w283 w285] -> w279
                  frame "Lakeshore335" {
                  }
                  frame "VersaLab", Default {
                    n95 = stacked-sequence {
                      tunnel: [w297] -> w288
                      tunnel: [w353] -> w285
                      tunnel: w287 -> [w290]
                      tunnel: w286 -> [w352]
                      tunnel: w289 -> [w299]
                      frame #0 {
                        n96 = Concatenate Strings("," ("字符串"), " " ("字符串")) -> (w309:string)
                        n97 = Fract/Exp String To Number(string=w290, offset=16 ("偏移量")) -> (offset past number=w349:i32, number=w301:dbl)  [unwired: 2 in]
                        n98 = Match Pattern(string=w290, regular expression=w309) -> (after substring=w351:string)  [unwired: 1 in, 3 out]
                        n99 = Match Pattern(string=w290, regular expression="or reverse" ("正则表达式")) -> (offset past match=w292:i32)  [unwired: 1 in, 3 out]
                        n100 = Match Pattern(string=w351, regular expression=w309) -> (after substring=w325:string)  [unwired: 1 in, 3 out]
                        n101 = Match Pattern(string=w290, regular expression="Step Delay ") -> (after substring=w296:string)  [unwired: 1 in, 3 out]
                        n102 = Add(x=w349, y=6) -> (x+y=w348:i32)
                        n103 = case shown="0, 默认" w292 {
                          tunnel: [TRUE ("Or Reserve?") FALSE ("Or Reserve?")] -> w291
                          frame 0, Default {
                          }
                          frame -1 {
                          }
                        }
                        n104 = Fract/Exp String To Number(string=w296) -> (number=w295:dbl)  [unwired: 3 in, 1 out]
                        n105 = Fract/Exp String To Number(string=w290, offset=w348) -> (offset past number=w330:i32, number=w302:dbl)  [unwired: 2 in]
                        n106 = Match Pattern(string=w325, regular expression=w309) -> (before substring=w324:string, after substring=w310:string)  [unwired: 1 in, 2 out]
                        n107 = Match Pattern(string=w310, regular expression=w309) -> (before substring=w308:string, after substring=w307:string)  [unwired: 1 in, 2 out]
                        n108 = Concatenate Strings("Un" ("字符串"), "H*" ("字符串"), "H^" ("字符串"), "1/" ("字符串"), "lo" ("字符串")) -> (w316:string)
                        n109 = Add(x=w330, y=6) -> (x+y=w328:i32)
                        n110 = call "string front part.vi"("字符串"=w324, "偏移量(0)"=2) -> ("result string"=w322:string)  [unwired: 9 in]
                        n111 = Match Pattern "spacing"(string=w316, regular expression=w322) -> (offset past match=w315:i32)  [unwired: 1 in, 3 out]
                        n112 = Fract/Exp String To Number(string=w290, offset=w328) -> (offset past number=w311:i32, number=w300:dbl)  [unwired: 2 in]
                        n113 = Concatenate Strings("P" ("字符串"), "O" ("字符串")) -> (w335:string)
                        n114 = Concatenate Strings("L" ("字符串"), "N" ("字符串"), "O" ("字符串"), "S" ("字符串")) -> (w341:string)
                        n115 = call "string front part.vi"("字符串"=w308, "偏移量(0)"=1) -> ("result string"=w345:string)  [unwired: 9 in]
                        n116 = call "string front part.vi"("字符串"=w307, "偏移量(0)"=1) -> ("result string"=w338:string)  [unwired: 9 in]
                        n117 = Match Pattern "Approach"(string=w341, regular expression=w345) -> (offset past match=w306:i32)  [unwired: 1 in, 3 out]
                        n118 = Match Pattern "Mode"(string=w335, regular expression=w338) -> (offset past match=w334:i32)  [unwired: 1 in, 3 out]
                        n119 = Divide(x=w315, y=2) -> (x/y=w313:dbl)
                        n120 = Add(x=w311, y=10) -> (x+y=w326:i32)
                        n121 = Fract/Exp String To Number(string=w290, offset=w326) -> (number=w303:dbl)  [unwired: 2 in, 1 out]
                        n122 = Subtract(x=w313, y=1.0) -> ()  [unwired: 1 out]
                        n123 = Subtract(x=w334, y=1) -> (x-y=w304:i32)
                        n124 = Subtract(x=w306, y=1) -> (x-y=w298:i32)
                        n125 = case shown="0, 默认" w298 {
                          tunnel: w304 -> [w362 w375]
                          tunnel: w298 -> [w364 _]
                          tunnel: w303 -> [w365 w377]
                          tunnel: w302 -> [w367 w374]
                          tunnel: w301 -> [w360 w376]
                          tunnel: w300 -> [w361 w373]
                          tunnel: w299 -> [w363 w378]
                          tunnel: w352 -> [w357 w371]
                          tunnel: [w358 w372] -> w297
                          tunnel: w295 -> [w366 _]
                          tunnel: [w356 w370] -> w353
                          tunnel: w291 -> [_ w369]
                          frame 0, Default {
                            n126 = call "setpoint(SubVI).vi"("Filed 2"=w367, "输出簇 2"=w357, "Delay"=w366, "steps number"=w365, "Approach"=w364, "Field"=w360, "type"=enum16{"temp", "field", "position"}."field" ("类型"), "Rate/speed"=w361, "Mode"=w362, "data"=w363) -> ("错误输出"=w358:errorcluster, "输出簇"=w356:T1)  [unwired: 8 in]
                          }
                          frame 3 {
                            n127 = call "sweep(SubVI).vi"("data"=w378, "类型"=set_type."field", "Or Reverse?"=w369, "steps number"=w377, "簇"=w371, "Field"=w376, "Mode"=w375, "Field 2"=w374, "Rate、speed"=w373) -> ("输出簇"=w370:T1, "错误输出"=w372:errorcluster)  [unwired: 5 in]
                          }
                        }
                      }
                    }
                  }
                }
              }
              frame "Select " {
                n128 = call "Select ch str (SubVI).vi"("字符串"=w382, "config"=w381) -> ("config out"=w380:T1)  [unwired: 9 in]
              }
              frame "Auto Ra" {
                n129 = call "Auto Range(SR830).vi"("error in (no error)"=w383, "簇"=w384) -> ()  [unwired: 9 in, 1 out]
              }
              frame "Wait Fo" {
                n130 = call "Wait For (str) (SubVI).vi"("簇"=w387, "字符串"=w389, "error in"=errorcluster {"status"=FALSE, "code"=0, "source"=""} ("error out")) -> ("错误输出"=w386:errorcluster)  [unwired: 7 in]
              }
              frame "Set Dat" {
                n131 = Unbundle By Name(w392) -> ("Instrument.genarl.数据文件"=w391:refnum<vi>)
                n132 = call "Set Data (str) (子VI).vi"("元素"=w392, "字符串"=w394) -> ("错误输出"=w393:errorcluster, "path"=w390:path)  [unwired: 8 in]
                n133 = property class="Path"(reference=w391, "Val(Sgnl)"=w390) -> ()  [unwired: 1 in, 2 out]
              }
              frame "End Seq" {
                n134 = Unbundle By Name(w396) -> ("Instrument.genarl.Aborting"=w395:refnum<vi>)
                n135 = property on="属性节点" class="Bool (严格)"(reference=w395, "Val(Sgnl)"=TRUE ("Abort")) -> ()  [unwired: 1 in, 2 out]
              }
              frame "Initial" {
                n136 = call "Initalize (seq）(SubVI).vi"("字符串"=w402, "簇"=w399) -> ("输出簇"=w401:T1)  [unwired: 9 in]
              }
              frame "Scan PZ" {
                n137 = Match Pattern(string=w404, regular expression="in" ("正则表达式")) -> (after substring=w408:string)  [unwired: 1 in, 3 out]
                n138 = Match Pattern(string=w404, regular expression="to" ("正则表达式")) -> (after substring=w409:string)  [unwired: 1 in, 3 out]
                n139 = Match Pattern(string=w404, regular expression="from" ("正则表达式")) -> (after substring=w414:string)  [unwired: 1 in, 3 out]
                n140 = Fract/Exp String To Number(string=w414, default (0 dbl)=0) -> (number=w407:i32)  [unwired: 2 in, 1 out]
                n141 = Fract/Exp String To Number(string=w409, default (0 dbl)=0) -> (number=w406:i32)  [unwired: 2 in, 1 out]
                n142 = Fract/Exp String To Number(string=w408, default (0 dbl)=0) -> (number=w405:i32)  [unwired: 2 in, 1 out]
                n143 = call "setpoint(SubVI).vi"("Filed 2"=w406, "输出簇 2"=w419, "steps number"=w405, "Field"=w407, "type"=set_type."PZT", "list?"=FALSE, "data"=w403) -> ("错误输出"=w417:errorcluster, "输出簇"=w418:T1)  [unwired: 11 in]
              }
              frame "Scan RP" {
                n144 = Match Pattern(string=w434, regular expression="interval" ("正则表达式")) -> (after substring=w442:string)  [unwired: 1 in, 3 out]
                n145 = Match Pattern(string=w434, regular expression="at" ("正则表达式")) -> (after substring=w431:string)  [unwired: 1 in, 3 out]
                n146 = Match Pattern(string=w434, regular expression="to" ("正则表达式")) -> (after substring=w436:string)  [unwired: 1 in, 3 out]
                n147 = Match Pattern(string=w434, regular expression="from" ("正则表达式")) -> (after substring=w443:string)  [unwired: 1 in, 3 out]
                n148 = Fract/Exp String To Number(string=w443, default (0 dbl)=0) -> (number=w426:i32)  [unwired: 2 in, 1 out]
                n149 = Fract/Exp String To Number(string=w436, default (0 dbl)=0) -> (number=w425:i32)  [unwired: 2 in, 1 out]
                n150 = Fract/Exp String To Number(string=w431, default (0 dbl)=0) -> (number=w430:i32)  [unwired: 2 in, 1 out]
                n151 = Fract/Exp String To Number(string=w442, default (0 dbl)=0) -> (number=w424:i32)  [unwired: 2 in, 1 out]
                n152 = Bundle By Name(cluster=w433, "StrainCell.slew(V/s)"=w430) -> (w429:T1)
                n153 = Unbundle By Name(w429) -> ("Instrument.325 for test.quantum design"=w428:refnum<k24>)
                n154 = call "GetTemperature.vi"("Instrument Ref In"=w428) -> ("Temperature"=w427:dbl)  [unwired: 4 in, 4 out]
                n155 = call "get v list.vi"("temp"=w427, "increase"=w424, "end"=w425, "begin"=w426) -> ("输出数组"=w423:dbl[])  [unwired: 7 in]
                n156 = call "setpoint(SubVI).vi"("输出簇 2"=w429, "type"=set_type."StrainCell", "list"=w423, "list?"=TRUE, "data"=w441) -> ("错误输出"=w439:errorcluster, "输出簇"=w440:T1)  [unwired: 13 in]
              }
              frame "Set RP1" {
                n157 = call "set RP100 voltage.vi"("error in (no error)"=w449, "字符串 2"=w453, "config"=w452) -> ("error out"=w450:errorcluster, "输出簇"=w451:T1)  [unwired: 7 in]
              }
              frame "Scan Ti" {
                n158 = Match Pattern(string=w464, regular expression="in " ("正则表达式")) -> (after substring=w455:string)  [unwired: 1 in, 3 out]
                n159 = Match Pattern(string=w464, regular expression="Time " ("正则表达式")) -> (after substring=w459:string)  [unwired: 1 in, 3 out]
                n160 = Fract/Exp String To Number(string=w459) -> (number=w458:dbl)  [unwired: 3 in, 1 out]
                n161 = Fract/Exp String To Number(string=w455, default (0 dbl)=0) -> (number=w457:i32)  [unwired: 2 in, 1 out]
                n162 = call "scan time(SubVI).vi"("total time"=w458, "config"=w463, "steps number"=w457, "data"=w465) -> ("输出簇"=w462:T1, "错误输出"=w461:errorcluster)  [unwired: 10 in]
              }
              frame "Delta d" {
                n163 = call "Delta delay (seq) (SubVI).vi"("字符串"=w468, "config"=w467) -> ("错误输出"=w466:errorcluster)  [unwired: 9 in]
              }
              frame "Delta r" {
                n164 = call "Delta range (seq) (SubVI).vi"("字符串"=w471, "config"=w470) -> ("错误输出"=w469:errorcluster)  [unwired: 9 in]
              }
              frame "Scan Po" {
                n165 = Unbundle By Name(w473) -> ("Instrument.genarl.Instrument Type"=w475:T5)
                n166 = case shown="\"VersaLab\", 默认" w475 {
                  tunnel: w477 -> [w482 _ w532]
                  tunnel: w476 -> [w481 _ w534]
                  tunnel: [w480 errorcluster {"status"=FALSE, "code"=0, "source"=""} ("错误输出") w530] -> w472
                  tunnel: w473 -> [w479 w528 w533]
                  tunnel: [w478 w528 w531] -> w474
                  frame "PPMS", "PPMS-Rotate" {
                    n167 = stacked-sequence {
                      tunnel: [w483] -> w480
                      tunnel: [w508] -> w478
                      tunnel: w482 -> [w493]
                      tunnel: w479 -> [w507]
                      tunnel: w481 -> [w485]
                      frame #0 {
                        n168 = Match Pattern(string=w493, regular expression="Sweep" ("正则表达式")) -> (match substring=w494:string)  [unwired: 1 in, 3 out]
                        n169 = Match Pattern(string=w493, regular expression="from " ("正则表达式")) -> (after substring=w490:string)  [unwired: 1 in, 3 out]
                        n170 = Match Pattern(string=w493, regular expression="Delay " ("正则表达式")) -> (after substring=w491:string)  [unwired: 1 in, 3 out]
                        n171 = Fract/Exp String To Number "dekay"(string=w491) -> (number=w488:dbl)  [unwired: 3 in, 1 out]
                        n172 = Fract/Exp String To Number "1"(string=w490) -> (offset past number=w505:i32, number=w484:dbl)  [unwired: 3 in]
                        n173 = Add(x=w505, y=4) -> (x+y=w503:i32)
                        n174 = Fract/Exp String To Number "2"(string=w490, offset=w503) -> (offset past number=w502:i32, number=w489:dbl)  [unwired: 2 in]
                        n175 = Add(x=w502, y=2) -> (x+y=w500:i32)
                        n176 = Fract/Exp String To Number "speed"(string=w490, offset=w500) -> (offset past number=w499:i32, number=w486:dbl)  [unwired: 2 in]
                        n177 = Add(x=w499, y=5) -> (x+y=w497:i32)
                        n178 = Fract/Exp String To Number "step"(use system decimal point (T)=TRUE ("使用系统小数点(T)"), string=w490, offset=w497) -> (number=w487:dbl)  [unwired: 1 in, 1 out]
                        n179 = case shown="\"Sweep\"" w494 {
                          tunnel: w489 -> [w518 w524]
                          tunnel: w488 -> [w515 _]
                          tunnel: w487 -> [w514 w526]
                          tunnel: w486 -> [w513 w523]
                          tunnel: w485 -> [w516 w527]
                          tunnel: w484 -> [w517 w525]
                          tunnel: [w512 w522] -> w483
                          tunnel: w507 -> [w511 w521]
                          tunnel: [w510 w520] -> w508
                          frame "假", Default {
                            n180 = call "setpoint(SubVI).vi"("Filed 2"=w518, "输出簇 2"=w511, "Delay"=w515, "steps number"=w514, "Field"=w517, "type"=set_type."position", "Rate/speed"=w513, "data"=w516) -> ("错误输出"=w512:errorcluster, "输出簇"=w510:T1)  [unwired: 10 in]
                          }
                          frame "Sweep" {
                            n181 = call "sweep(SubVI).vi"("data"=w527, "类型"=set_type."position" ("type"), "steps number"=w526, "簇"=w521, "Field"=w525, "Field 2"=w524, "Rate、speed"=w523) -> ("输出簇"=w520:T1, "错误输出"=w522:errorcluster)  [unwired: 7 in]
                          }
                        }
                      }
                    }
                  }
                  frame "VersaLab", Default {
                  }
                  frame "9T mag old" {
                    n182 = stacked-sequence {
                      tunnel: [w549] -> w530
                      tunnel: [w550] -> w531
                      tunnel: w532 -> [w553]
                      tunnel: w533 -> [w546]
                      tunnel: w534 -> [w551]
                      frame #0 {
                        n183 = Match Pattern(string=w553, regular expression="Position " ("正则表达式")) -> (after substring=w554:string)  [unwired: 1 in, 3 out]
                        n184 = Match Pattern(string=w553, regular expression="Delay " ("正则表达式")) -> (after substring=w538:string)  [unwired: 1 in, 3 out]
                        n185 = Fract/Exp String To Number "delay"(string=w538) -> (number=w545:dbl)  [unwired: 3 in, 1 out]
                        n186 = Match Pattern(string=w554, regular expression=" from " ("正则表达式")) -> (before substring=w555:string, after substring=w539:string)  [unwired: 1 in, 2 out]
                        n187 = case shown="\"out plane\", 默认" w555 {
                          tunnel: [enum16{"in plane", "out plane"}."out plane" ("轴向") enum16{"in plane", "out plane"}."in plane" ("轴向")] -> w556
                          frame "out plane", Default {
                          }
                          frame "in plane" {
                          }
                        }
                        n188 = Fract/Exp String To Number "1"(string=w539) -> (number=w547:dbl)  [unwired: 3 in, 1 out]
                        n189 = Match Pattern(string=w539, regular expression=" to " ("正则表达式")) -> (after substring=w557:string)  [unwired: 1 in, 3 out]
                        n190 = Fract/Exp String To Number "2"(string=w557) -> (number=w543:dbl)  [unwired: 3 in, 1 out]
                        n191 = Match Pattern(string=w557, regular expression="in " ("正则表达式")) -> (after substring=w542:string)  [unwired: 1 in, 3 out]
                        n192 = Fract/Exp String To Number "step"(string=w542) -> (number=w544:dbl)  [unwired: 3 in, 1 out]
                        n193 = call "setpoint(SubVI).vi"("Filed 2"=w543, "输出簇 2"=w546, "Delay"=w545, "steps number"=w544, "Field"=w547, "轴向"=w556, "type"=set_type."position", "Rate/speed"=1.0, "data"=w551) -> ("错误输出"=w549:errorcluster, "输出簇"=w550:T1)  [unwired: 9 in]
                      }
                    }
                  }
                }
              }
              frame "Move Sa" {
                n194 = Unbundle By Name(w560) -> ("Instrument.325 for test.quantum design"=w563:refnum<k24>, "Instrument.genarl.Instrument Type"=w562:T5)
                n195 = case shown="\"9T mag old\"" w562 {
                  tunnel: w564 -> [w568 _ w572]
                  tunnel: [w567 errorcluster {"status"=FALSE, "code"=0, "source"=""} ("错误输出") w573] -> w561
                  tunnel: w563 -> [_ _ _]
                  tunnel: w560 -> [w566 _ w571]
                  frame "PPMS-Rotate", "lengtou2" {
                    n196 = Unbundle By Name(w566) -> ("Instrument"=w565:T3)
                    n197 = call "Move to (SubVI).vi"("Instrument"=w565, "字符串"=w568) -> ("错误输出"=w567:errorcluster)  [unwired: 9 in]
                  }
                  frame Default {
                  }
                  frame "9T mag old" {
                    n198 = Unbundle By Name(w571) -> ("Instrument"=w570:T3)
                    n199 = call "Cmag Move to (SubVI).vi"("Instrument"=w570, "字符串"=w572) -> ("错误输出"=w573:errorcluster)  [unwired: 9 in]
                  }
                }
              }
              frame "Set Cur" {
                n200 = call "Set Current (seq) (SubVI).vi"("字符串"=w577, "config"=w576) -> ("输出簇"=w575:T1)  [unwired: 9 in]
              }
              frame "Scan Cu" {
                n201 = stacked-sequence {
                  tunnel: [w602] -> w578
                  tunnel: [w601] -> w580
                  tunnel: w581 -> [w590]
                  tunnel: w582 -> [w599]
                  tunnel: w579 -> [w600]
                  frame #0 {
                    n202 = Match Pattern(string=w590, regular expression="in " ("正则表达式")) -> (after substring=w591:string)  [unwired: 1 in, 3 out]
                    n203 = Match Pattern(string=w590, regular expression="from " ("正则表达式")) -> (offset past match=w595:i32)  [unwired: 1 in, 3 out]
                    n204 = Decimal String To Number(string=w591) -> (number=w598:i32)  [unwired: 2 in, 1 out]
                    n205 = Fract/Exp String To Number(string=w590, offset=w595) -> (offset past number=w593:i32, number=w587:dbl)  [unwired: 2 in]
                    n206 = Add(x=w593, y=5) -> (x+y=w594:i32)
                    n207 = Divide(x=w587, y=1000.0) -> (x/y=w586:dbl)
                    n208 = Fract/Exp String To Number(string=w590, offset=w594) -> (number=w585:dbl)  [unwired: 2 in, 1 out]
                    n209 = Divide(x=w585, y=1000.0) -> (x/y=w584:dbl)
                    n210 = call "setpoint(SubVI).vi"("Filed 2"=w584, "输出簇 2"=w600, "steps number"=w598, "Field"=w586, "type"=set_type."current", "data"=w599) -> ("错误输出"=w602:errorcluster, "输出簇"=w601:T1)  [unwired: 12 in]
                  }
                }
              }
              frame "Set Gat" {
                w615 = " " ("正则表达式")
                n211 = Match Pattern(string=w613, regular expression=w615) -> (after substring=w618:string)  [unwired: 1 in, 3 out]
                n212 = Match Pattern(string=w618, regular expression=w615) -> (after substring=w617:string)  [unwired: 1 in, 3 out]
                n213 = Fract/Exp String To Number(string=w617) -> (number=w605:dbl)  [unwired: 3 in, 1 out]
                n214 = Match Pattern(string=w617, regular expression=w615) -> (after substring=w616:string)  [unwired: 1 in, 3 out]
                n215 = Match Pattern(string=w616, regular expression=w615) -> (after substring=w614:string)  [unwired: 1 in, 3 out]
                n216 = Match Pattern(string=w614, regular expression=w615) -> (after substring=w606:string)  [unwired: 1 in, 3 out]
                n217 = Fract/Exp String To Number(string=w614) -> (number=w612:dbl)  [unwired: 3 in, 1 out]
                n218 = case shown="\"ChB\"" w606 {
                  tunnel: [w619 w620] -> w607
                  frame "ChB" {
                    w619 = 1 items=["Channel A", "Channel B"] ("Channel")
                  }
                  frame "ChA", Default {
                    w620 = 0 items=["Channel A", "Channel B"] ("Channel")
                  }
                }
                n219 = Unbundle By Name(w611) -> ("gating type"=w610:T7, "Instrument.genarl.Aborting"=w609:refnum<vi>)
                n220 = Unbundle By Name(w611) -> ("2614B.VISA"=w603:refnum<visa-resource-name>, "2400.VISA"=w604:refnum<visa-resource-name>)
                n221 = call "set gating.vi"("2400 VISA"=w604, "gating type"=w610, "Source Measure Unit Channel (0: Channel A)"=w607, "2614 VISA"=w603, "Voltage Level"=w605, "RATE(mV/s)"=w612, "abort"=w609) -> ("error out"=w608:errorcluster)  [unwired: 7 in, 1 out]
              }
              frame "Scan Ga" {
                n222 = flat-sequence {
                  tunnel: [w642] -> w630
                  tunnel: w632 -> [w649]
                  tunnel: [w637] -> w631
                  tunnel: [w636] -> w629
                  tunnel: [w635] -> w628
                  tunnel: [w634] -> w627
                  tunnel: [w633] -> w625
                  frame #0 {
                    n223 = Match Pattern(string=w649, regular expression="from " ("正则表达式")) -> (after substring=w647:string)  [unwired: 1 in, 3 out]
                    n224 = Fract/Exp String To Number(string=w647) -> (number=w634:dbl)  [unwired: 3 in, 1 out]
                    n225 = Match Pattern(string=w647, regular expression="to " ("正则表达式")) -> (after substring=w646:string)  [unwired: 1 in, 3 out]
                    n226 = Fract/Exp String To Number(string=w646) -> (number=w635:dbl)  [unwired: 3 in, 1 out]
                    n227 = Match Pattern(string=w646, regular expression="at " ("正则表达式")) -> (after substring=w644:string)  [unwired: 1 in, 3 out]
                    n228 = Fract/Exp String To Number(string=w644) -> (number=w633:dbl)  [unwired: 3 in, 1 out]
                    n229 = Match Pattern(string=w644, regular expression="in " ("正则表达式")) -> (after substring=w641:string)  [unwired: 1 in, 3 out]
                    n230 = Match Pattern(string=w641, regular expression=" steps, " ("正则表达式")) -> (after substring=w639:string)  [unwired: 1 in, 3 out]
                    n231 = Decimal String To Number(string=w641) -> (number=w642:i32)  [unwired: 2 in, 1 out]
                    n232 = Match Pattern(string=w639, regular expression=", Step Delay ") -> (before substring=w638:string, after substring=w652:string)  [unwired: 1 in, 2 out]
                    n233 = case shown="\"ChA\"" w638 {
                      tunnel: [w653 w654] -> w637
                      frame "ChB", Default {
                        w653 = 1 items=["ChA", "ChB"] ("Gating ch(2614)")
                      }
                      frame "ChA" {
                        w654 = 0 items=["ChA", "ChB"] ("Gating ch(2614)")
                      }
                    }
                    n234 = Fract/Exp String To Number(string=w652) -> (number=w636:dbl)  [unwired: 3 in, 1 out]
                  }
                }
                n235 = call "setpoint(SubVI).vi"("Filed 2"=w628, "输出簇 2"=w624, "Delay"=w629, "steps number"=w630, "Field"=w627, "Source Measure Unit Channel (0: Channel A)"=w631, "type"=enum16{"temp", "field", "position", "gating"}."gating" ("类型"), "Rate/speed"=w625, "data"=w623) -> ("错误输出"=w621:errorcluster, "输出簇"=w622:T1)  [unwired: 9 in]
              }
              frame "-1", Default {
              }
            }
          }
          frame "End Scan" {
          }
        }
      }
      frame True {
      }
    }
    n236 = flat-sequence {
      tunnel: w10 -> [w41]
      tunnel: w9 -> [w40]
      tunnel: w8 -> [_]
      frame #0 {
        n237 = property class="DigNum (严格)"(reference=w41, "Val(Sgnl)"=w40) -> ()  [unwired: 1 in, 2 out]
      }
    }
    n238 = Unbundle By Name(w33) -> ("Instrument.genarl.Aborting"=w23:refnum<vi>)
    n239 = case shown="错误" w8 {
      tunnel: w17 -> [_ w54]
      tunnel: w8 -> [_ w53]
      tunnel: w23 -> [_ w50]
      frame No Error {
      }
      frame Error {
        n240 = Unbundle By Name(w53) -> ("source"=w55:string)
        n241 = property on="属性节点" class="Bool (严格)"(reference=w50, "Val(Sgnl)"=TRUE) -> ()  [unwired: 1 in, 2 out]
        n242 = Concatenate Strings(w54, w55) -> (w52:string)
        n243 = Bundle(cluster=w53, "source"=w52) -> (w51:errorcluster)  [unwired: 2 in]
        n244 = call <vilib>:"General Error Handler.vi"("error in (no error)"=w51) -> ()  [unwired: 10 in, 5 out]
      }
    }
    n245 = property class="Bool (严格)"(reference=w23) -> ("Value"=w32:bool)  [unwired: 1 in, 2 out]
    n246 = Or(x=w37, y=w32) -> (x .or. y?=w35:bool)
    n247 = Or(x=w8, y=w35) -> (x .or. y?=w26:bool)
    n248 = Or(x=w27, y=w26) -> (x .or. y?=w25:bool)
  }
  "config out" <- w5
  "错误输出" <- w1
